vi "20211029_HW04.vi"() -> ()   [LabVIEW 2019]
panel:
  out "Avg.":dbl[](array[numeric])
  in  "Nums":dbl[](array[numeric])=[10.0, 20.0, 30.0, 40.0, 50.0, 60.0]
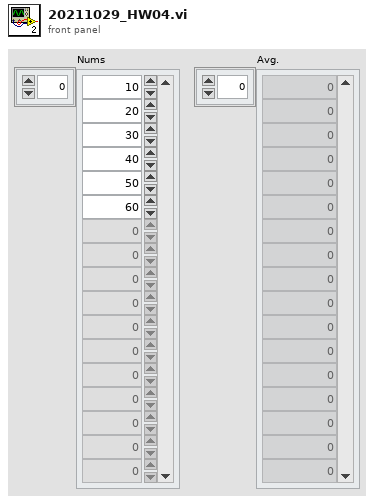
[diagram p1: front panel]
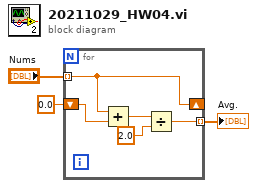
[diagram p0: block diagram]
diagram:
  n1 = for {
    tunnel: "Nums" -> [w8] mode=indexing
    shift-right: [w8] -> _
    shift-left: 0.0 ("Numeric") -> [w7]
    tunnel: [w4] -> w1 mode=indexing
    n2 = Add(x=w8, y=w7) -> (x+y=w6:dbl)
    n3 = Divide(x=w6, y=2.0) -> (x/y=w4:dbl)
  }
  "Avg." <- w1
